vi "Joystick Angle.vi"(10 "y":dbl, 11 "x":dbl) -> (2 "Angle":dbl)   [LabVIEW 2016]
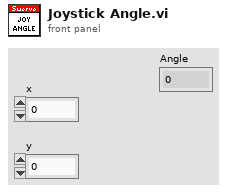
[diagram p1: front panel]
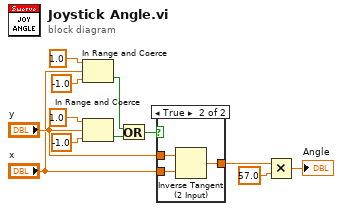
[diagram p0: block diagram]
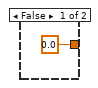
[diagram p2: hidden frame]
diagram:
  n1 = In Range and Coerce(upper limit=1.0, x="x", lower limit=-1.0) -> (In Range?=w8:bool)  [unwired: 1 out]
  n2 = In Range and Coerce(upper limit=1.0, x="y", lower limit=-1.0) -> (In Range?=w7:bool)  [unwired: 1 out]
  n3 = Or(x=w8, y=w7) -> (x .or. y?=w4:bool)
  n4 = case shown="True" w4 {
    tunnel: [0.0 w16] -> w12
    tunnel: "y" -> [_ w15]
    tunnel: "x" -> [_ w14]
    frame False {
    }
    frame True {
      n5 = Inverse Tangent (2 Input)(1:w14, 2:w15) -> (0:w16:dbl)
    }
  }
  n6 = Multiply(x=w12, y=57.0) -> (x*y=→"Angle":dbl)
